vi "Translation_Plus.vi"(9 "other Translation":T1, 11 "In Translation":T1) -> (3 "Out Translation":T1)   [LabVIEW 2019, in "Trajectory_Library.lvlib"]
doc: "Adds two translations in 2d space and returns the sum. This is similar to vector addition.\n \nFor example, Translation2d{1.0, 2.5} + Translation2d{2.0, 5.5} = Translation2d{3.0, 8.0}\n\nParameters:\n - IN Translation - This translation data structure\n - other Translation - The translation data structure to add\n\nReturns\n - Out Translation - The summation of the two translations."
uses:
  Trajectory_Library.lvlib
  TRANSLATION2D.ctl
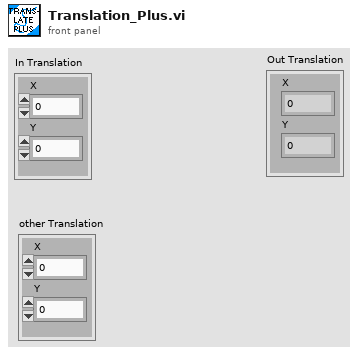
[diagram p1: front panel]
types:
  T1 = typedef "Trajectory_Library.lvlib/TRANSLATION2D.ctl" = cluster{"X":dbl, "Y":dbl}
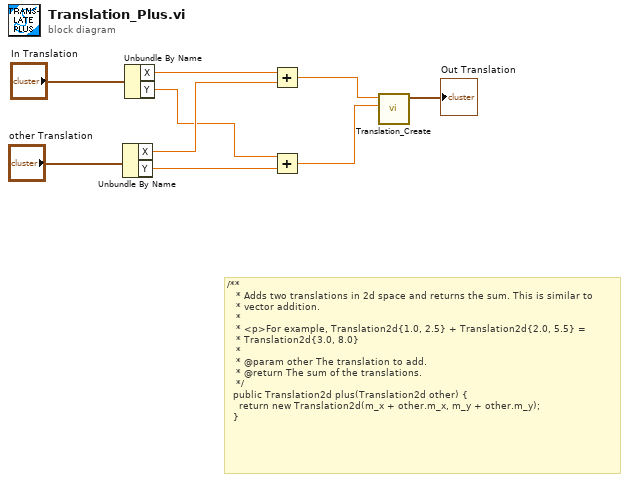
[diagram p0: block diagram]
diagram:
  # "/**\n   * Adds two translations in 2d space and returns the sum. This is similar to\n   * vector addition.\n   *\n   * <p>For example, Translation2d{1.0, 2.5} + Translation2d{2.0, 5.5} =\n   * Translation2d{3.0, 8.0}\n   *\n   * @param other The translation to add.\n   * @return The sum of the translations.\n   */\n  public Translation2d plus(Translation2d other) {\n    return new Translation2d(m_x + other.m_x, m_y + other.m_y);\n  }"
  n1 = Unbundle By Name("other Translation") -> ("X"=w6:dbl, "Y"=w5:dbl)
  n2 = Unbundle By Name("In Translation") -> ("X"=w7:dbl, "Y"=w4:dbl)
  n3 = Add(x=w7, y=w6) -> (x+y=w3:dbl)
  n4 = Add(x=w4, y=w5) -> (x+y=w2:dbl)
  n5 = call "Translation_Create.vi"("Y"=w2, "X"=w3) -> ("TRANSLATION"=→"Out Translation":T1)  [unwired: 9 in]
